vi "Prompting the user.vi"   [LabVIEW 2015]
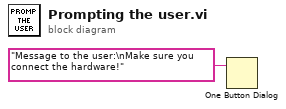
[diagram p0: block diagram]
diagram:
  n1 = One Button Dialog(message="Message to the user:\nMake sure you connect the hardware!") -> ()  [unwired: 1 in, 1 out]
